vi "Sucesion 2.vi"() -> ()   [LabVIEW 2017]
panel:
  out "Número":i64
  out "Iteración":i64
  # "SUCESIÓN 2"
  # "Cecilia Nuñez\n   11541028"
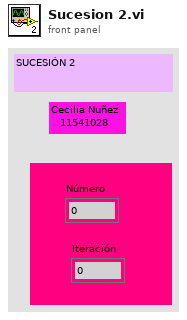
[diagram p1: front panel]
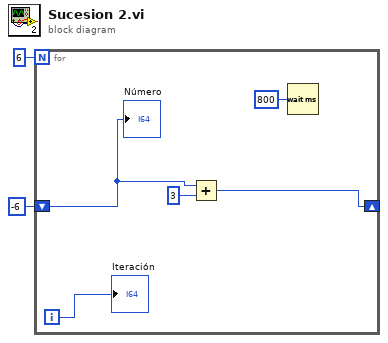
[diagram p0: block diagram]
diagram:
  n1 = for {
    N: 6 -> [_]
    shift-right: [w6] -> _
    shift-left: i64 -6 -> [w5]
    i -> [w4]
    n2 = Add(x=w5, y=i64 3) -> (x+y=w6:i64)
    n3 = Wait (ms)(milliseconds to wait=u32 800) -> ()  [unwired: 1 out]
    "Número" <- w5
    "Iteración" <- w4
  }
